vi "Database Type.vi"(8 "error in":errorcluster, 11 "DB Type":u16) -> (0 "error out":errorcluster, 3 "DB Type":u16)   [LabVIEW 2014]
doc: "<B>Copyrights</B>: (c) MHWirth 2015. All rights reserved.\n\nThis subVI sets the csv file delimeter."
panel:
  in  "Text Ring":u16(ring) items=["Excel"=0, "CSV"=2]
  in  "update":bool
  # "Database Type"
  # "Set the type of database that\nis created using this application."
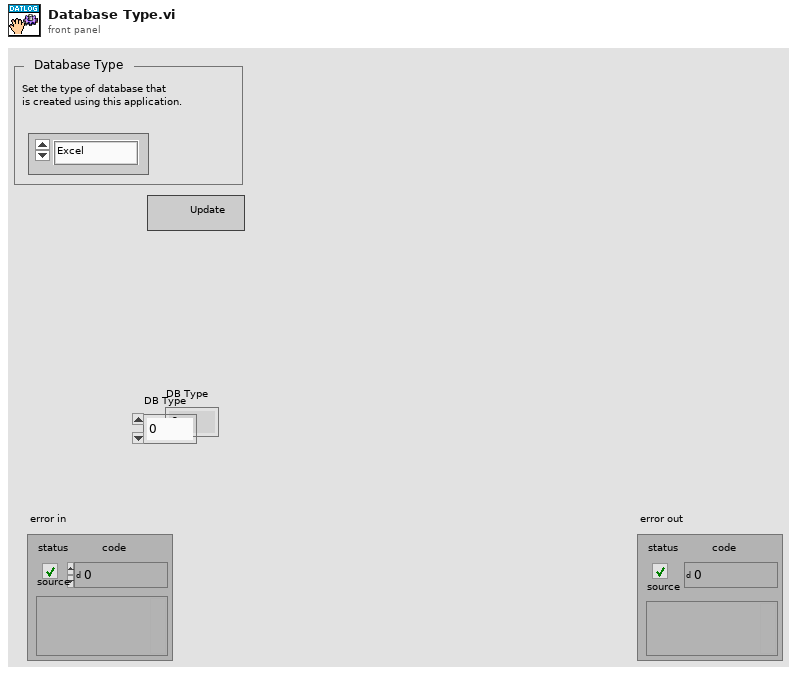
[diagram p1: front panel]
types:
  T1 = typedef "eventvkey.ctl" = enum16{"ASCII", "Enter", "Return", "Shift", "Ctrl", "Alt", "Cmd", "Opt", "Caps", "NumLock", "Clear", "Break", "Up", "Down", "Left", "Right", "Insert", "Delete", "Home", "End", "PageUp", "PageDown", "Escape", "Help", "Pause", "ScrollLock", "F1", "F2", "F3", "F4", "F5", "F6", "F7", "F8", "F9", "F10", "F11", "F12", "F13", "F14", "F15", "F16", "F17", "F18", "F19", "F20", "F21", "F22", "F23", "F24", "Play", "VolumeUp", "VolumeDown", "Mute", "Two Byte Char"}
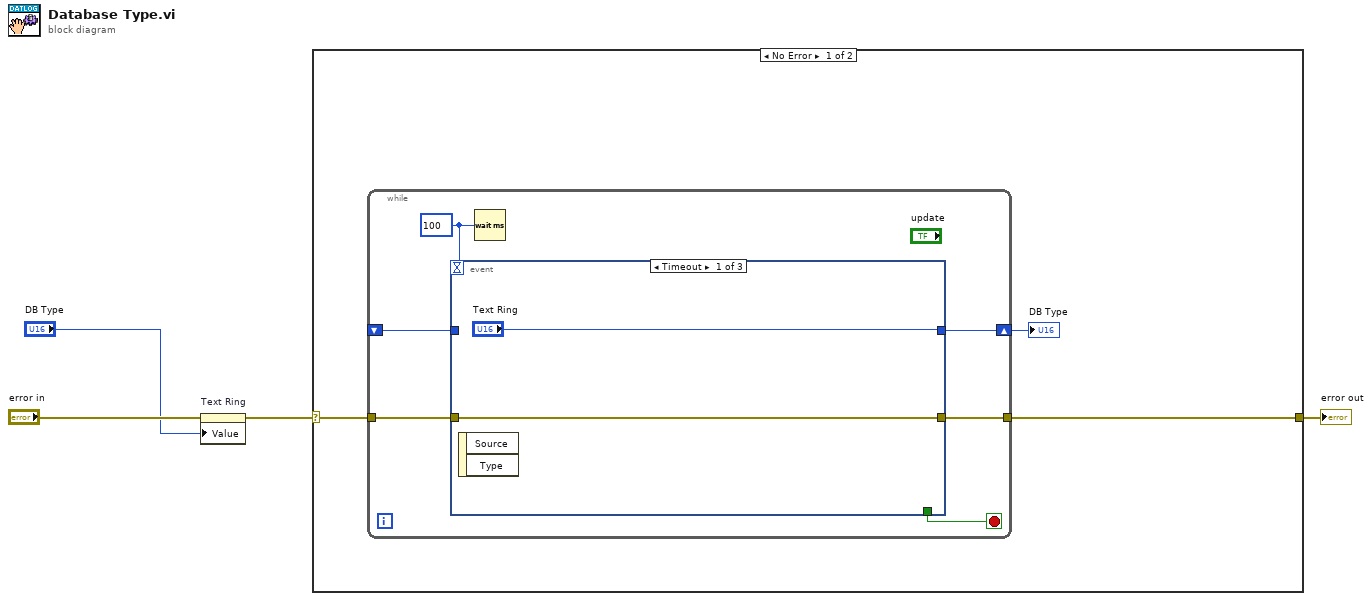
[diagram p0: block diagram]
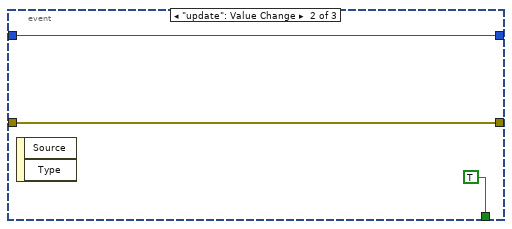
[diagram p2: hidden frame]
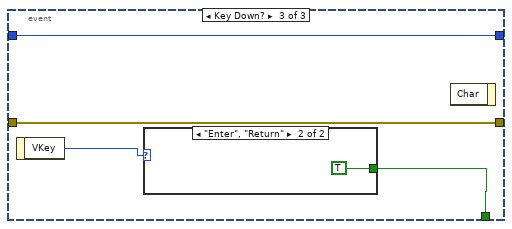
[diagram p3: hidden frame]
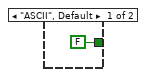
[diagram p4: hidden frame]
diagram:
  n1 = property on="Text Ring" class="Ring (strict)"(error in="error in", "Value"="DB Type") -> (error out=w3:errorcluster)  [unwired: 1 in, 1 out]
  n2 = case shown="No Error" w3 {
    selector: w3 -> [w7 w25]
    tunnel: [w6 w25] -> w4
    frame No Error {
      n3 = while {
        shift-right: [w11] -> w5
        shift-left: _ -> [w13]
        tunnel: w7 -> [w9]
        tunnel: [w8] -> w6
        stop <- w10 stop-if-true
        w12 = u32 100 ("milliseconds to wait")
        n4 = event shown="[0] Timeout" {
          selector: _ -> [_ _ _]
          dyn-events: _ -> [_ _ _]
          timeout: w12 -> [_ _ _]
          tunnel: w13 -> [_ w17 w21]
          tunnel: ["Text Ring" w17 w21] -> w11
          tunnel: [_ TRUE w20] -> w10
          tunnel: w9 -> [w14 w16 w22]
          tunnel: [w14 w16 w22] -> w8
          event Timeout {
            n5 = event-data() -> ()  [unwired: 1 in, 2 out]
          }
          event "update": Value Change {
            n6 = event-data() -> ()  [unwired: 1 in, 2 out]
          }
          event Key Down? {
            n7 = event-data() -> ("VKey"=w19:T1)  [unwired: 1 in]
            n8 = case shown="\"Enter\", \"Return\"" w19 {
              tunnel: [FALSE TRUE] -> w20
              frame "ASCII", Default {
              }
              frame "Enter", "Return" {
              }
            }
            n9 = event-data() -> ()  [unwired: 2 in, 1 out]
          }
        }
        n10 = Wait (ms)(milliseconds to wait=w12) -> ()  [unwired: 1 out]
      }
      "DB Type" <- w5
    }
    frame Error {
    }
  }
  "error out" <- w4
